vi "Move_Arm_to_Camera2.vi"(8 "error in":errorcluster, 10 "Desired Height":dbl=150.0 format="%#_13g", 11 "Machine In":refnum<visa-resource-name>) -> (0 "Z Coordinate":dbl=5.0, 1 "Y Coordinate":dbl, 2 "X Coordinate":dbl, 3 "Machine Out":refnum<visa-resource-name>, 4 "error out":errorcluster)   [LabVIEW 2018]
doc: "Example interface for controlling uArm Swift Pro."
panel:
  in  "Write Buffer":string="G90 G0 X1\n"
  out "read buffer":string
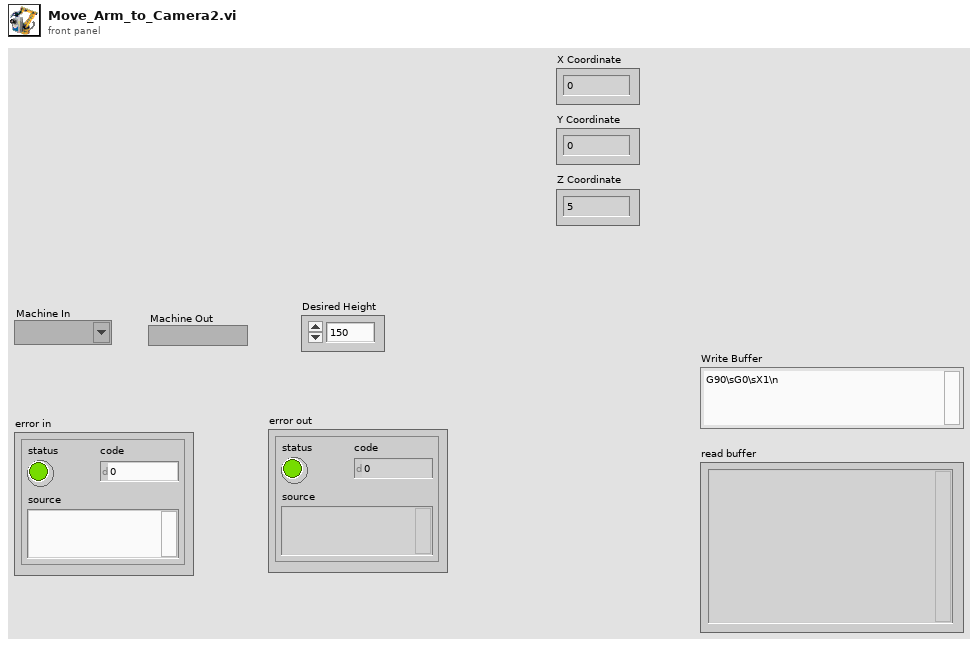
[diagram p1: front panel]
types:
  T1 = cluster{"Numeric Control":dbl, "Numeric Control":dbl}[]
  T2 = cluster{"Numeric Control":dbl, "Numeric Control":dbl}
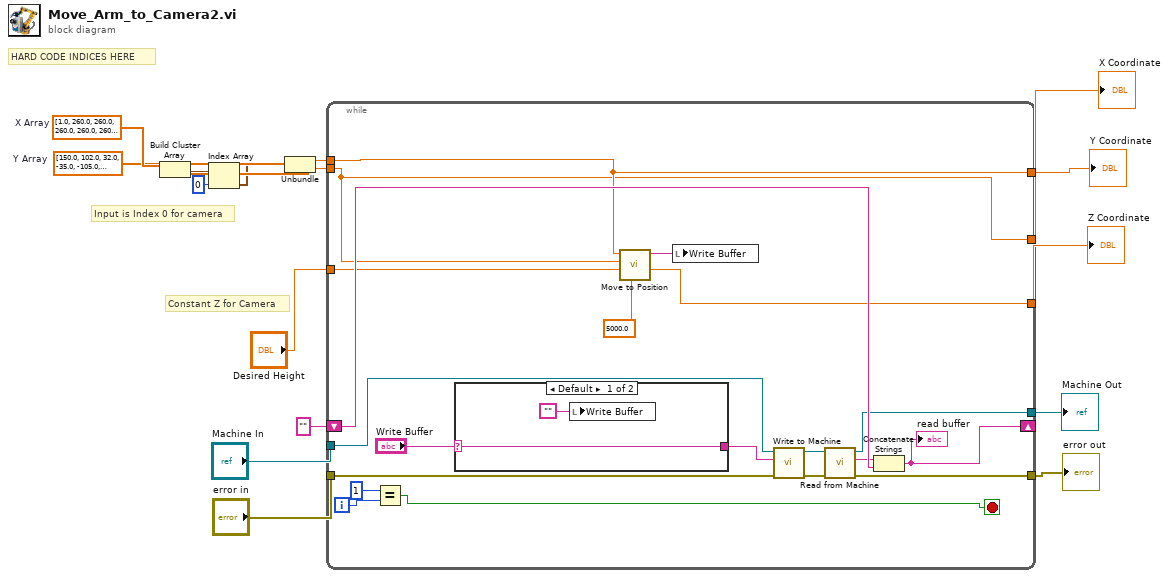
[diagram p0: block diagram]
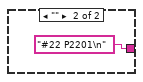
[diagram p2: hidden frame]
diagram:
  w14 = dbl[] [150.0, 102.0, 32.0, -35.0, -105.0, -175.0, 172.0, 102.0, 32.0, -35.0, -105.0, -175.0, 172.0, 102.0, 32.0, -35.0, -105.0, -175.0]  # Y Array
  w15 = dbl[] [1.0, 260.0, 260.0, 260.0, 260.0, 260.0, 180.0, 180.0, 180.0, 180.0, 180.0, 180.0, 105.0, 105.0, 105.0, 105.0, 105.0, 105.0]  # X Array
  # "Constant Z for Camera"
  # "HARD CODE INDICES HERE"
  # "Input is Index 0 for camera"
  n1 = Build Cluster Array(w15, w14) -> (w13:T1)
  n2 = Index Array(array=w13, index=0) -> (element=w12:T2)
  n3 = Unbundle(w12) -> ("Numeric Control"=w10:dbl, "Numeric Control"=w11:dbl)
  n4 = while {
    tunnel: "Machine In" -> [w33]
    tunnel: "error in" -> [w30]
    shift-right: [w31] -> _
    shift-left: "" -> [w32]
    tunnel: [w29] -> w7
    tunnel: [w25] -> w6
    tunnel: w11 -> [w18]
    tunnel: w10 -> [w19]
    tunnel: [w19] -> w5
    tunnel: [w18] -> w4
    tunnel: [w17] -> w3
    tunnel: "Desired Height" -> [w17]
    i -> [w22]
    stop <- w20 stop-if-true
    n5 = Equal?(x=1, y=w22) -> (x = y?=w20:bool)
    n6 = case shown="Default" "Write Buffer" {
      selector: "Write Buffer" -> [w37 _]
      tunnel: [w37 "#22 P2201\n"] -> w34
      frame Default {
        n7 = local write "Write Buffer"("") -> ()
      }
      frame "" {
      }
    }
    n8 = call "Move to Position.vi"("Speed"=5000.0, "Z-Position"=w17, "Y-Position"=w18, "X-Position"=w19) -> ("G-Code String"=w24:string)  [unwired: 7 in]
    n9 = local write "Write Buffer"(w24) -> ()
    n10 = call "Write to Machine .vi"("error in (no error)"=w30, "G-Code String In"=w34, "Machine In"=w33) -> ("error out"=w27:errorcluster, "Machine Out"=w26:refnum<visa-resource-name>)  [unwired: 7 in]
    n11 = call "Read from Machine.vi"("error in (no error)"=w27, "Machine In"=w26) -> ("error out"=w25:errorcluster, "read buffer"=w28:string, "Machine Out"=w29:refnum<visa-resource-name>)  [unwired: 7 in]
    n12 = Concatenate Strings(w28, w32) -> (w31:string)
    "read buffer" <- w31
  }
  "Machine Out" <- w7
  "error out" <- w6
  "Y Coordinate" <- w5
  "X Coordinate" <- w4
  "Z Coordinate" <- w3
